vi "Frequency (Half Cycle).vi"(0 "waveform":waveform(dbl), 1 "reset? (F)":bool, 5 "zero crossing":dbl[](array[numeric]), 7 "samples since the last cross":dbl[](array[numeric]), 9 "system info in":refnum<class "EP System Info.lvclass">, 11 "error in (no error)":errorcluster, 12 "voltage flag? (F)":bool) -> (4 "one-cycle frequency":T1, 6 "half-cycle frequency":T1, 8 "averaged frequency":dbl format="%#_9g", 10 "system info out":refnum<class "EP System Info.lvclass">, 15 "error out":errorcluster)   [LabVIEW 2014, in "NI_EP_Power Quality.lvlib"]
doc: "Calculates the half, single, and 10/12-cycle frequency of a voltage or current waveform, by using the zero crossings. You can use the Zero Crossing VI to calculate <B>zero crossing</B> and <B>samples since the last cross</B>. This VI refreshes the half and single-cycle frequency every half-cycle. If the value is flagged, this VI returns the last non-flagged frequency. You can use <B>half-cycle frequency</B> with the 10 Seconds instance of the EN50160 Aggregation VI to calculate frequencies according to IEC 61000-4-30:2008.\n\nThis VI supports measuring one channel on one line at one time."
uses:
  <vilib>/addons/Electrical Power/PQ/NI_EP_Power Quality.lvlib
  <vilib>/addons/Electrical Power/PQ/Common/Classes/System Info/EP System Info.lvclass
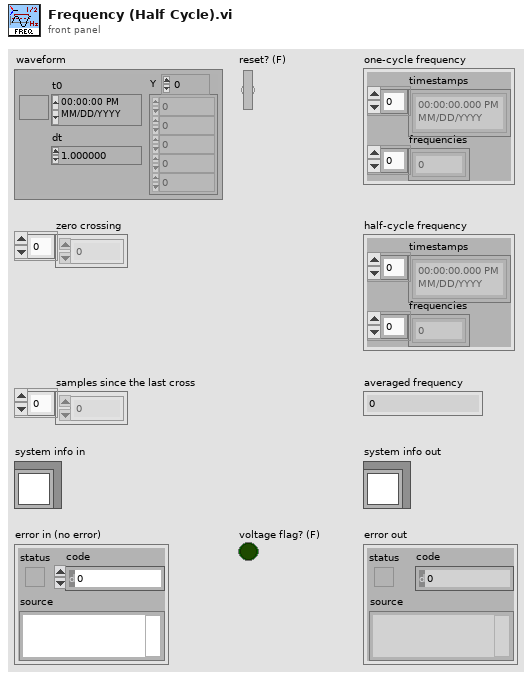
[diagram p1: front panel]
types:
  T1 = cluster{"timestamps":timestamp[], "frequencies":dbl[]}
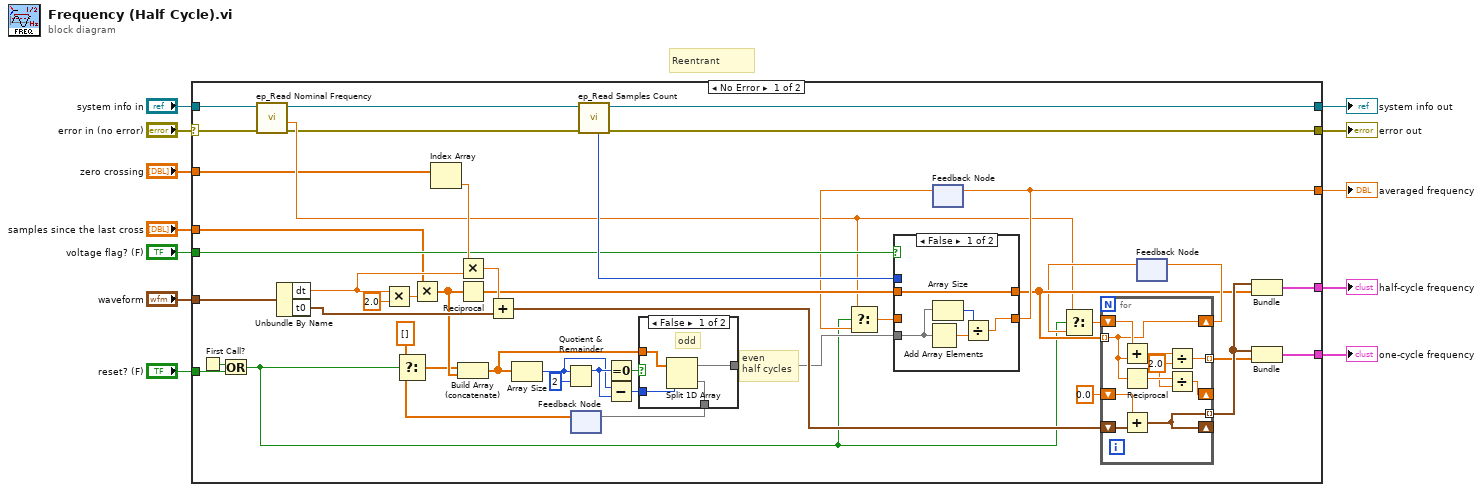
[diagram p0: block diagram]
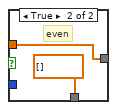
[diagram p2: hidden frame]
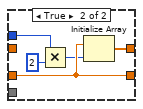
[diagram p3: hidden frame]
diagram:
  # "Reentrant"
  n1 = case shown="No Error" "error in (no error)" {
    selector: "error in (no error)" -> [w57 w86]
    tunnel: "system info in" -> [w58 w87]
    tunnel: "waveform" -> [w54 _]
    tunnel: [w41 w87] -> w9
    tunnel: [w28 w86] -> w8
    tunnel: [w53 _] -> w7
    tunnel: [w56 _] -> w6
    tunnel: [w55 _] -> w5
    tunnel: "voltage flag? (F)" -> [w39 _]
    tunnel: "reset? (F)" -> [w19 _]
    tunnel: "zero crossing" -> [w16 _]
    tunnel: "samples since the last cross" -> [w15 _]
    frame No Error {
      # "even\nhalf cycles"
      n2 = First Call?() -> (First Call?: T/F=w17:bool)
      n3 = Or(x=w17, y=w19) -> (x .or. y?=w18:bool)
      n4 = call <vilib>:"ep_Read Nominal Frequency.vi"("error in (no error)"=w57, "system info in"=w58) -> ("error out"=w13:errorcluster, "nominal frequency value"=w20:dbl, "system info out"=w14:refnum<class "EP System Info.lvclass">)  [unwired: 6 in, 1 out]
      n5 = Unbundle By Name(w54) -> ("dt"=w38:dbl, "t0"=w59:timestamp)
      n6 = Multiply(x=w38, y=2.0) -> (x*y=w48:dbl)
      n7 = Multiply(x=w15, y=w48) -> (x*y=w29:dbl[])
      n8 = Index Array(array=w16) -> (element=w47:dbl)  [unwired: 1 in]
      n9 = Multiply(x=w47, y=w38) -> (x*y=w46:dbl)
      n10 = Reciprocal(x=w29) -> (1/x=w43:dbl[])
      n11 = Add(x=w46, y=w59) -> (x+y=w45:timestamp)
      n12 = feedback #1() -> (w26:dbl[])  [unwired: 1 in]
      n13 = Select(t=dbl[] [], s=w18, f=w26) -> (s? t:f=w27:dbl[])
      n14 = Build Array (concatenate)(w27, w29) -> (w35:dbl[])
      n15 = Array Size(array=w35) -> (size(s)=w32:i32)
      n16 = Quotient & Remainder(x=w32, y=2) -> (x-y*floor(x/y)=w33:i32)  [unwired: 1 out]
      n17 = call <vilib>:"ep_Read Samples Count.vi"("error in (no error)"=w13, "system info in"=w14) -> ("error out"=w28:errorcluster, "system info out"=w41:refnum<class "EP System Info.lvclass">, "cycles per interval"=w40:i32)  [unwired: 5 in, 2 out]
      n18 = Equal To 0?(x=w33) -> (x = 0?=w34:bool)
      n19 = Subtract(x=w32, y=w33) -> (x-y=w31:i32)
      n20 = case shown="False" w34 {
        tunnel: [w63 dbl[] []] -> w36
        tunnel: w35 -> [w62 w64]
        tunnel: [w61 w64] -> w30
        tunnel: w31 -> [w60 _]
        frame False {
          # "odd"
          n21 = Split 1D Array(array=w62, index=w60) -> (first subarray=w61:dbl[], second subarray=w63:dbl[])
        }
        frame True {
          # "even"
        }
      }
      n22 = feedback-in #1(w36) -> ()
      n23 = feedback #2() -> (w23:dbl)  [unwired: 1 in]
      n24 = Select(t=w20, s=w18, f=w23) -> (s? t:f=w24:dbl)
      n25 = case shown="False" w39 {
        tunnel: [w78 w85] -> w42
        tunnel: w43 -> [w78 _]
        tunnel: w40 -> [_ w82]
        tunnel: w24 -> [_ w84]
        tunnel: [w76 w84] -> w53
        tunnel: w30 -> [w77 _]
        frame False {
          n26 = Add Array Elements(numeric array=w77) -> (sum=w79:dbl)
          n27 = Array Size(array=w77) -> (size(s)=w80:i32)
          n28 = Divide(x=w80, y=w79) -> (x/y=w76:dbl)
        }
        frame True {
          n29 = Multiply(x=w82, y=2) -> (x*y=w81:i32)
          n30 = Initialize Array(w84, w81) -> (w85:dbl[])
        }
      }
      n31 = feedback-in #2(w53) -> ()
      n32 = feedback #3() -> (w21:dbl)  [unwired: 1 in]
      n33 = Select(t=w20, s=w18, f=w21) -> (s? t:f=w22:dbl)
      n34 = for {
        tunnel: [w70] -> w52 mode=indexing
        tunnel: w42 -> [w72] mode=indexing
        shift-right: [w72] -> w50
        shift-left: w22 -> [w75]
        tunnel: [w73] -> w49 mode=indexing
        shift-right: [w70] -> _
        shift-left: w45 -> [w69]
        shift-right: [w67] -> _
        shift-left: 0.0 -> [w66]
        w68 = 2.0 ("y")
        n35 = Add(x=w75, y=w72) -> (x+y=w74:dbl)
        n36 = Reciprocal(x=w72) -> (1/x=w71:dbl)
        n37 = Add(x=w66, y=w69) -> (x+y=w70:timestamp)
        n38 = Divide(x=w74, y=w68) -> (x/y=w73:dbl)
        n39 = Divide(x=w71, y=w68) -> (x/y=w67:dbl)
      }
      n40 = feedback-in #3(w50) -> ()
      n41 = Bundle(w52, w42) -> (w56:cluster{timestamp[], dbl[]})  [unwired: 1 in]
      n42 = Bundle(w52, w49) -> (w55:cluster{timestamp[], dbl[]})  [unwired: 1 in]
    }
    frame Error {
    }
  }
  "error out" <- w8
  "one-cycle frequency" <- w5
  "averaged frequency" <- w7
  "system info out" <- w9
  "half-cycle frequency" <- w6
